vi "Packer. 1_U32 to U64.vi"(7 "Swap I16 Numbers":bool=TRUE, 8 "Data Valid":bool, 11 "Input Data":u32) -> (0 "Data Valid":bool, 3 "Output Data (Packed U64)":u64)   [LabVIEW 2011]
uses:
  <vilib>/rvi/FXPMathLib/basic elements/FxpDiscreteDelay/XNode/nifxpmath_DiscreteDelay.xnode
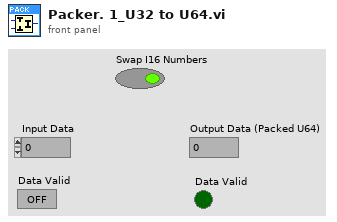
[diagram p1: front panel]
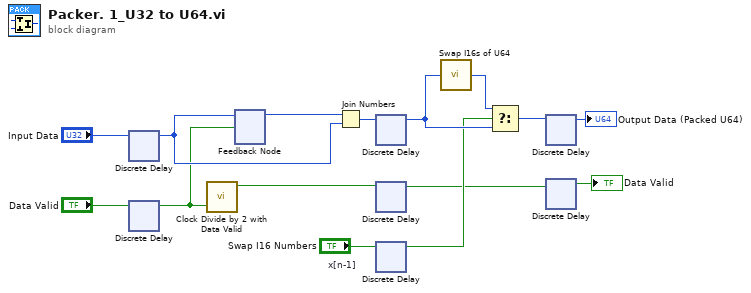
[diagram p0: block diagram]
diagram:
  n1 = xnode "Discrete Delay"("D"="Input Data") -> ("Q"=w14:u32)
  n2 = xnode "Discrete Delay"("D"="Data Valid") -> ("Q"=w12:bool)
  n3 = call <userlib>:"Clock Divide by 2 with Data Valid.vi"("Data Valid"=w12) -> ("CLK/2"=w13:bool)  [unwired: 10 in]
  n4 = feedback #1 "x[n-1]"() -> (w15:u32)  [unwired: 1 in]
  n5 = feedback-in #1(w14, w12) -> ()
  n6 = Join Numbers(hi=w15, lo=w14) -> ((hi.lo)=w9:u64)
  n7 = xnode "Discrete Delay"("D"=w9) -> ("Q"=w8:u64)
  n8 = xnode "Discrete Delay"("D"=w13) -> ("Q"=w5:bool)
  n9 = xnode "Discrete Delay"("D"="Swap I16 Numbers") -> ("Q"=w6:bool)
  n10 = call <userlib>:"Swap I16s of U64.vi"("Number"=w8) -> ("swapped number"=w10:u64)  [unwired: 14 in]
  n11 = Select(t=w10, s=w6, f=w8) -> (s? t:f=w11:u64)
  n12 = xnode "Discrete Delay"("D"=w11) -> ("Q"=→"Output Data (Packed U64)":u64)
  n13 = xnode "Discrete Delay"("D"=w5) -> ("Q"=→"Data Valid":bool)
